vi "Find Control Reference By Name.vi"(8 "error in (no error)":errorcluster, 10 "Name":string, 11 "Controls[]":refnum<vi>[](array[refnum])) -> (0 "error out":errorcluster, 3 "Ctl Refnum":refnum<vi>)   [LabVIEW 2011, in "Simple Error Out.xctl"]
uses:
  Simple Error Out.xctl
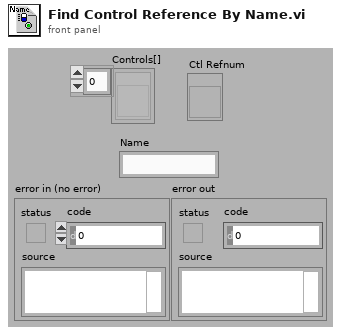
[diagram p1: front panel]
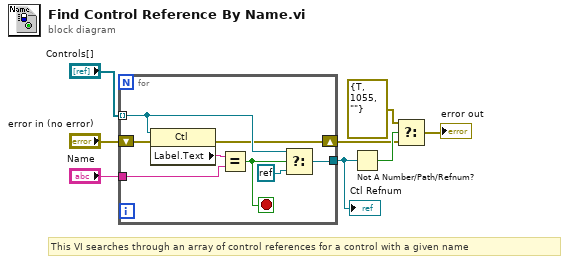
[diagram p0: block diagram]
diagram:
  # "This VI searches through an array of control references for a control with a given name"
  n1 = for {
    tunnel: "Controls[]" -> [w14] mode=indexing
    tunnel: "Name" -> [w15]
    tunnel: [w12] -> w5
    shift-right: [w9] -> w3
    shift-left: "error in (no error)" -> [w10]
    stop <- w11 stop-if-true
    n2 = property class="Ctl"(reference=w14, error in=w10) -> (error out=w9:errorcluster, "Label.Text"=w16:string)  [unwired: 1 out]
    n3 = Equal?(x=w16, y=w15) -> (x = y?=w11:bool)
    n4 = Select(t=w14, s=w11, f=refnum<k0> refnum) -> (s? t:f=w12:refnum<vi>)
  }
  "Ctl Refnum" <- w5
  n5 = Not A Number/Path/Refnum?(number/path/refnum=w5) -> (NaN/Path/Refnum?=w4:bool)
  n6 = Select(t=errorcluster {"status"=TRUE, "code"=1055, "source"=""}, s=w4, f=w3) -> (s? t:f=→"error out":errorcluster)
